vi "sample_ControlFilterWheels.vi"() -> ()   [LabVIEW 2012]
panel:
  in  "Goto Position 2":i32
  out "Connected 2":bool
  in  "Goto Position":i32
  out "Connected":bool
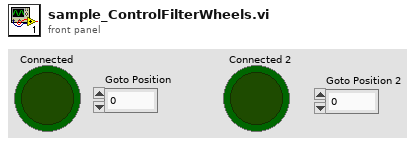
[diagram p1: front panel]
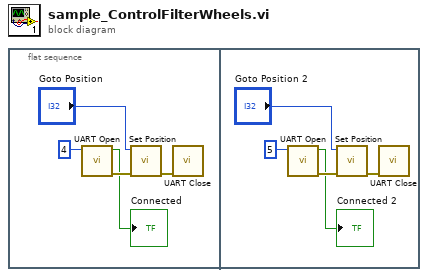
[diagram p0: block diagram]
diagram:
  n1 = flat-sequence {
    frame #0 {
      n2 = call "UART Open.vi"("Serial Port"=4) -> ("error out"=w3:errorcluster, "Success?"=→"Connected":bool)  [unwired: 9 in]
      n3 = call "Set Position.vi"("error in (no error)"=w3, "Position"="Goto Position") -> ("error out"=w2:errorcluster)  [unwired: 9 in]
      n4 = call "UART Close.vi"("error in (no error)"=w2) -> ()  [unwired: 10 in, 1 out]
    }
    frame #1 {
      n5 = call "UART Open.vi"("Serial Port"=5) -> ("error out"=w8:errorcluster, "Success?"=→"Connected 2":bool)  [unwired: 9 in]
      n6 = call "Set Position.vi"("error in (no error)"=w8, "Position"="Goto Position 2") -> ("error out"=w7:errorcluster)  [unwired: 9 in]
      n7 = call "UART Close.vi"("error in (no error)"=w7) -> ()  [unwired: 10 in, 1 out]
    }
  }
